vi "poly_control_value_from_name_self_multi.vi"(8 "error in (no error)":errorcluster, 9 "control names":string[](array[string])) -> (0 "error out":errorcluster, 1 "Values":variant[](array[variant]), 4 "found?":bool[](array[boolean]), 5 "ctrl refs":refnum<vi>[](array[refnum]))   [LabVIEW 2015]
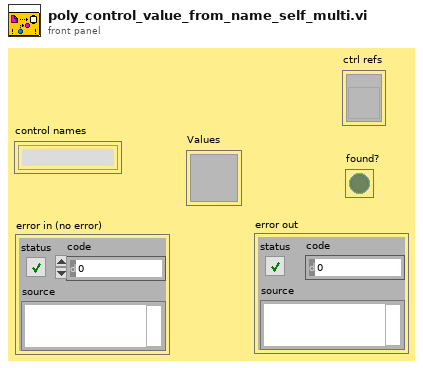
[diagram p1: front panel]
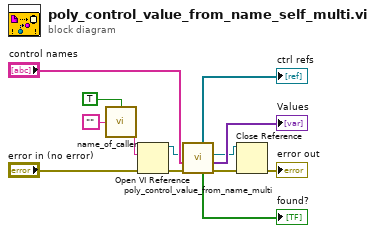
[diagram p0: block diagram]
diagram:
  n1 = call "name_of_caller.vi"("is in inlined vi? (F)"=TRUE, "name of caller in"="") -> ("name of caller out"=w3:string)  [unwired: 2 in]
  n2 = Open VI Reference(vi path=w3, error in (no error)="error in (no error)") -> (vi reference=w7:refnum<vi>, error out=w5:errorcluster)  [unwired: 4 in]
  n3 = call "poly_control_value_from_name_multi.vi"("error in (no error)"=w5, "control names"="control names", "vi ref"=w7) -> ("error out"=w9:errorcluster, "Values"=→"Values":variant[], "vi ref dup"=w8:refnum<vi>, "found?"=→"found?":bool[], "ctrl refs"=→"ctrl refs":refnum<vi>[])  [unwired: 4 in]
  n4 = Close Reference(reference=w8, error in (no error)=w9) -> (error out=→"error out":errorcluster)
